vi "Send Set Render Prio.vi"(7 "Message Priority (Normal)":T2=enum."Normal", 8 "error in (no error)":errorcluster, 10 "Low Prio Rendering":T1, 11 "Message Enqueuer":refnum<class "Message Enqueuer.lvclass">) -> (0 "error out":errorcluster, 3 "Message Enqueuer out":refnum<class "Message Enqueuer.lvclass">)   [LabVIEW 2020, in "Signal Analysis.lvlib" / "Set Render Prio Msg.lvclass"]
doc: "This VI sends the message to an actor."
uses:
  Set Render Prio Msg.lvclass
  <vilib>/ActorFramework/Message Enqueuer/Message Enqueuer.lvclass
  <vilib>/ActorFramework/Message Enqueuer/Message Priority.ctl
  Signal Analysis/Low Prio Rendering.ctl
  C:/Program Files/National Instruments/LabVIEW 2025/vi.lib/ActorFramework/Message/Message.lvclass
  Set Render Prio Msg.lvclass/Set Render Prio Msg.ctl
  <vilib>/ActorFramework/Message Enqueuer/Message Enqueuer.lvclass/Message Enqueuer.ctl
  <vilib>/ActorFramework/Message Priority Queue/Priority Enqueue.vi
  Signal Analysis/Signal Analysis.lvclass
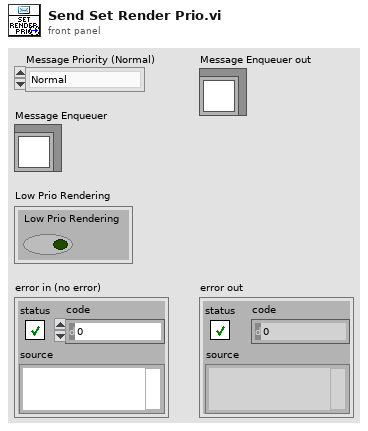
[diagram p1: front panel]
types:
  T1 = typedef "Signal Analysis.lvlib/Signal Analysis.lvclass/Low Prio Rendering.ctl" = cluster{"Low Prio Rendering":bool}
  T2 = typedef "Actor Framework.lvlib/Message Enqueuer.lvclass/Message Priority.ctl" = enum16{"Low", "Normal", "High"}
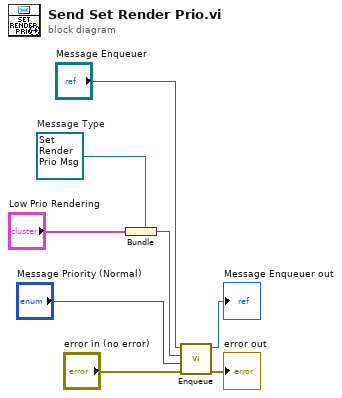
[diagram p0: block diagram]
diagram:
  w5 = refnum<class "Set Render Prio Msg.lvclass"> refnum  # Message Type
  n1 = Bundle(cluster=w5, "Low Prio Rendering") -> (w4:refnum<class "Set Render Prio Msg.lvclass">)
  n2 = call <vilib>:"Enqueue.vi"("error in (no error)"="error in (no error)", "Message Priority (Normal)"="Message Priority (Normal)", "Message"=w4, "Message Enqueuer in"="Message Enqueuer") -> ("error out"=→"error out":errorcluster, "Message Enqueuer out"=→"Message Enqueuer out":refnum<class "Message Enqueuer.lvclass">)  [unwired: 6 in]
